vi "BuildResPDU.vi"(7 "从站IP":u32=3232236289 format="%08x", 8 "Node RX":bool[][](array[boolean]), 9 "Node RWr":i16[][](array[numeric])=[[0, 0, 0, 0, 0, 0, 0, 0, 0, 0, 0, 0, 0, 0, 0, 0, 0, 0, 0, 0, 0, 0, 0, 0, 0, 0, 0, 0, 0, 0, 0, 0], [0, 0, 0, 0, 0, 0, 0, 0, 0, 0, 0, 0, 0, 0, 0, 0, 0, 0, 0, 0, 0, 0, 0, 0, 0, 0, 0, 0, 0, 0, 0, 0], [0, 0, 0, 0, 0, 0, 0, 0, 0, 0, 0, 0, 0, 0, 0, 0, 0, 0, 0, 0, 0, 0, 0, 0, 0, 0, 0, 0, 0, 0, 0, 0], [0, 0, 0, 0, 0, 0, 0, 0, 0, 0, 0, 0, 0, 0, 0, 0, 0, 0, 0, 0, 0, 0, 0, 0, 0, 0, 0, 0, 0, 0, 0, 0]] format="%04x", 10 "占用站数":i32=4, 11 "主站信息":T1={"主站IP"=3232236538, "组号"=1, "帧号"=28198, "时间戳"=1532683204396} {"时间戳" format="%016x"; "帧号" format="%04x"; "主站IP" format="%08x"}) -> (0 "输出字符串":string, 3 "主站IP":u32 format="%08x")   [LabVIEW 2018]
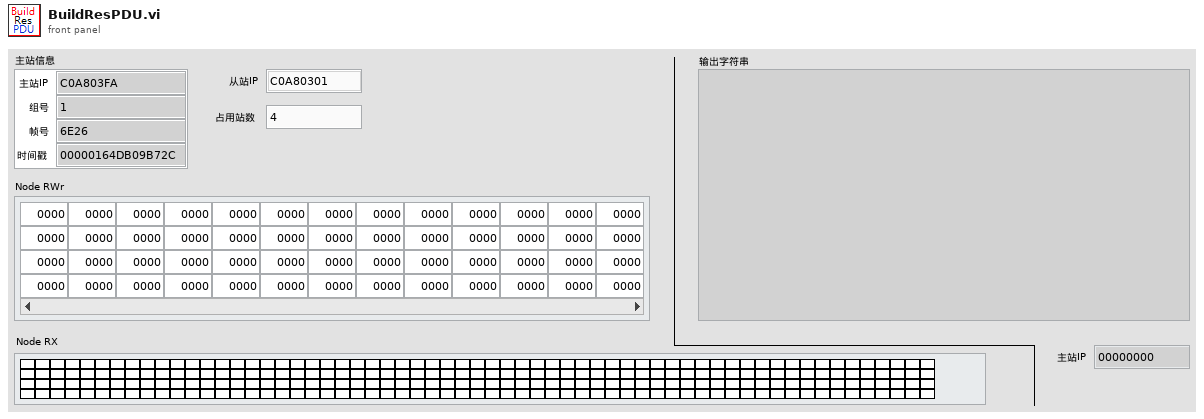
[diagram p1: front panel]
types:
  T1 = cluster{"主站IP":u32, "组号":u8, "帧号":u16, "时间戳":u64}
  T2 = enum16{"big-endian, network order", "native, host order", "little-endian"}
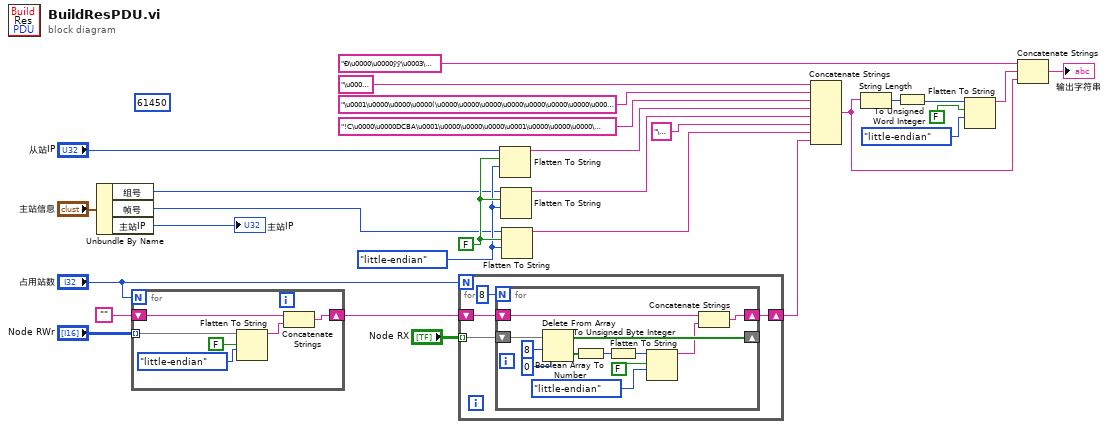
[diagram p0: block diagram]
diagram:
  w12 = T2."little-endian" ("字节顺序(0:big-endian, network order)")
  w13 = FALSE ("预置数组或字符串大小？ (T)")
  (unwired) u32 61450 ("地址")
  n1 = Unbundle By Name("主站信息") -> ("组号"=w5:u8, "帧号"=w4:u16, "主站IP"=→"主站IP":u32)
  n2 = for {
    N: "占用站数" -> [_]
    tunnel: "Node RWr" -> [w32] mode=indexing
    shift-right: [w29] -> w26
    shift-left: "" -> [w31]
    n3 = Flatten To String(anything=w32, prepend array or string size? (T)=FALSE ("预置数组或字符串大小？ (T)"), byte order (0:big-endian, network order)=T2."little-endian" ("字节顺序(0:big-endian, network order)")) -> (data string=w30:string)  [unwired: 1 in, 2 out]
    n4 = Concatenate Strings(w31, w30) -> (w29:string)
  }
  n5 = for {
    N: "占用站数" -> [_]
    tunnel: "Node RX" -> [w37] mode=indexing
    shift-right: [w35] -> w7
    shift-left: w26 -> [w36]
    n6 = for {
      N: 8 -> [_]
      shift-right: [w47] -> _
      shift-left: w37 -> [w50]
      shift-right: [w43] -> w35
      shift-left: w36 -> [w42]
      n7 = Delete From Array(array=w50, length=8 ("长度"), index=0 ("索引")) -> (deleted portion=w46:bool[], array with subset deleted=w47:bool[])
      n8 = Boolean Array To Number(Boolean array=w46) -> (number=w40:u32)
      n9 = To Unsigned Byte Integer(number=w40) -> (unsigned 8bit integer=w39:u8)
      n10 = Flatten To String(anything=w39, prepend array or string size? (T)=FALSE ("预置数组或字符串大小？ (T)"), byte order (0:big-endian, network order)=T2."little-endian" ("字节顺序(0:big-endian, network order)")) -> (data string=w41:string)  [unwired: 1 in, 2 out]
      n11 = Concatenate Strings(w42, w41) -> (w43:string)
    }
  }
  n12 = Flatten To String(anything="从站IP", prepend array or string size? (T)=w13, byte order (0:big-endian, network order)=w12) -> (data string=w11:string)  [unwired: 1 in, 2 out]
  n13 = Flatten To String(anything=w5, prepend array or string size? (T)=w13, byte order (0:big-endian, network order)=w12) -> (data string=w10:string)  [unwired: 1 in, 2 out]
  n14 = Flatten To String(anything=w4, prepend array or string size? (T)=w13, byte order (0:big-endian, network order)=w12) -> (data string=w8:string)  [unwired: 1 in, 2 out]
  n15 = Concatenate Strings("\u0000\u0000", "\u0001\u0000\u0000\u0000(\u0000\u0000\u0000\u0000\u0000\u0000\u0000\u0000\u0000\u0000\u0000\u0000\u0000\u0000\u0000", "!C\u0000\u0000DCBA\u0001\u0000\u0000\u0000\u0001\u0000\u0000\u0000\u0000\u0000\u0000\u0000", w11, w10, "\u0000", w8, w7) -> (w16:string)
  n16 = String Length(string=w16) -> (length=w22:i32)
  n17 = To Unsigned Word Integer(number=w22) -> (unsigned 16bit integer=w20:u16)
  n18 = Flatten To String(anything=w20, prepend array or string size? (T)=FALSE ("预置数组或字符串大小？ (T)"), byte order (0:big-endian, network order)=T2."little-endian" ("字节顺序(0:big-endian, network order)")) -> (data string=w17:string)  [unwired: 1 in, 2 out]
  n19 = Concatenate Strings("Ð\u0000\u0000ÿÿ\u0003\u0000", w17, w16) -> (→"输出字符串":string)
